vi "Untitled 1.vi"() -> ()   [LabVIEW 2015]
uses:
  Scanning Software_Demokritos_2015_v7/libs/XGL_DPP.lvlib
panel:
  out "x != 0?":bool
  in  "DPP Configuration":T1={"reset_recovery_time"=300, "edge_peaking_time"=4, "flat_top"=7, "peaking_time"=32, "gain"=1.0, "max_risetime"=0.0, "fast_filter_thr"=45, "zero_peak_freq"=1.0, "inverted_input"=0, "base_offset"=0, "reset_threshold"=1000, "overflow_recovery"=0, "tail_coefficient"=0.0, "energy_filter_thr"=23, "energy_baseline_thr"=23, "max_peaking_time"=35, "edge_flat_top"=1, "time_constant"=0.0, "baseline_samples"=64, "other_param"=0}
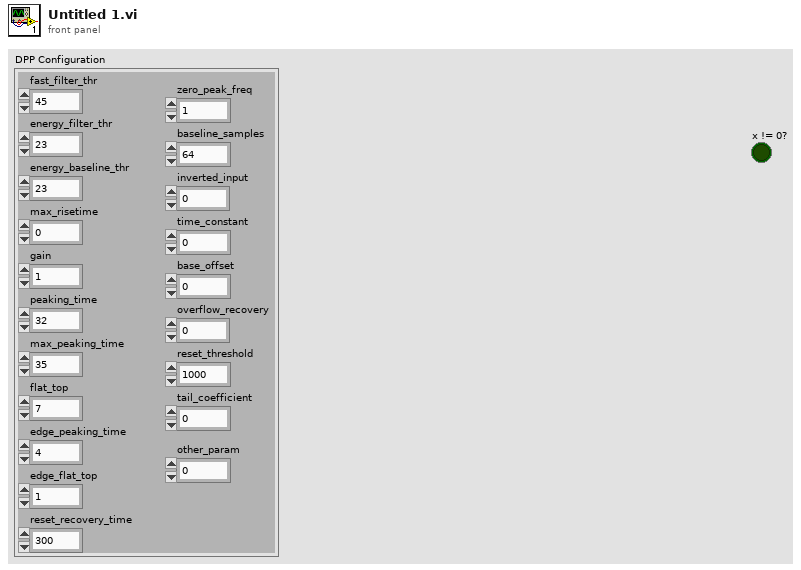
[diagram p1: front panel]
types:
  T1 = cluster{"reset_recovery_time":u32, "edge_peaking_time":u32, "flat_top":u32, "peaking_time":u32, "gain":dbl, "max_risetime":dbl, "fast_filter_thr":u32, "zero_peak_freq":dbl, "inverted_input":u8, "base_offset":u32, "reset_threshold":u32, "overflow_recovery":u32, "tail_coefficient":dbl, "energy_filter_thr":u32, "energy_baseline_thr":u32, "max_peaking_time":u32, "edge_flat_top":u32, "time_constant":dbl, "baseline_samples":u32, "other_param":u32}
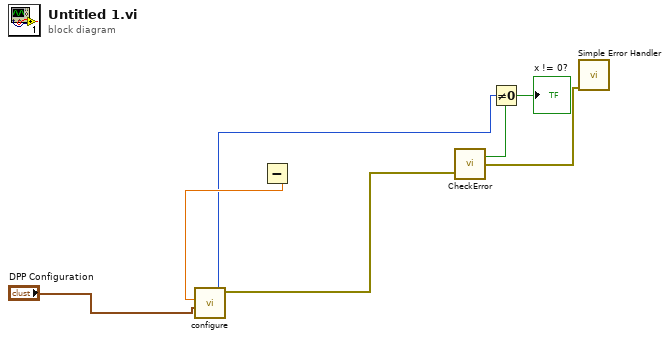
[diagram p0: block diagram]
diagram:
  n1 = Subtract() -> (x=w6:dbl, y=w1:dbl, x-y=w9:dbl)
  n2 = call "configure.vi"("DPP Configuration"="DPP Configuration", "Board"=w9) -> ("function return"=w7:u32, "error out"=w8:errorcluster, "error in (no error)"=w4:errorcluster, "identifier"=w5:string)  [unwired: 2 in]
  n3 = Not Equal To 0?(x=w7) -> (x != 0?=w10:bool)
  "x != 0?" <- w10
  n4 = call "CheckError.vi"("error in (no error)"=w8, "ret_val"=w10) -> ("error out"=w3:errorcluster)
  n5 = call <vilib>:"Simple Error Handler.vi"("error in (no error)"=w3) -> ()  [unwired: 4 in, 5 out]
